vi "Calculate Intersection Circles.vi"(6 "r2":dbl, 7 "r1":dbl, 8 "d":dbl, 9 "c":dbl, 10 "b":dbl, 11 "a":dbl) -> (0 "y2":dbl, 1 "x2":dbl, 2 "y1":dbl, 3 "x1":dbl)   [LabVIEW 2014, in "Position.lvclass"]
uses:
  Position.lvclass
panel:
  out "k":dbl
  out "p":dbl
  out "f":dbl
  out "e":dbl
  # "Usage:\n(a, b) signifies the (x, y) coordinates of circle 1 with radius r1.\n(c, d) signifies the (x, y) coordinates of circle 2 with radius r2.\n\nThe VI will return 4 values:\n- (x, y) coordinates where / if the circles intersect, as x1 and y1.\n- (x, y) coordinates where / if the circles intersect secondly, as x2 and y2.\n\nImportant: if the circles do not intersect 'NaN' will be returned"
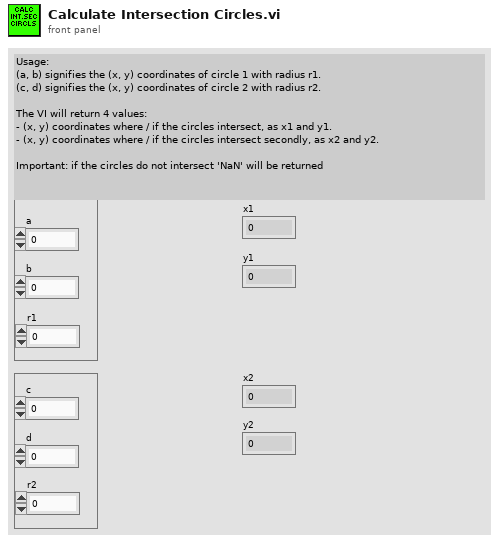
[diagram p1: front panel]
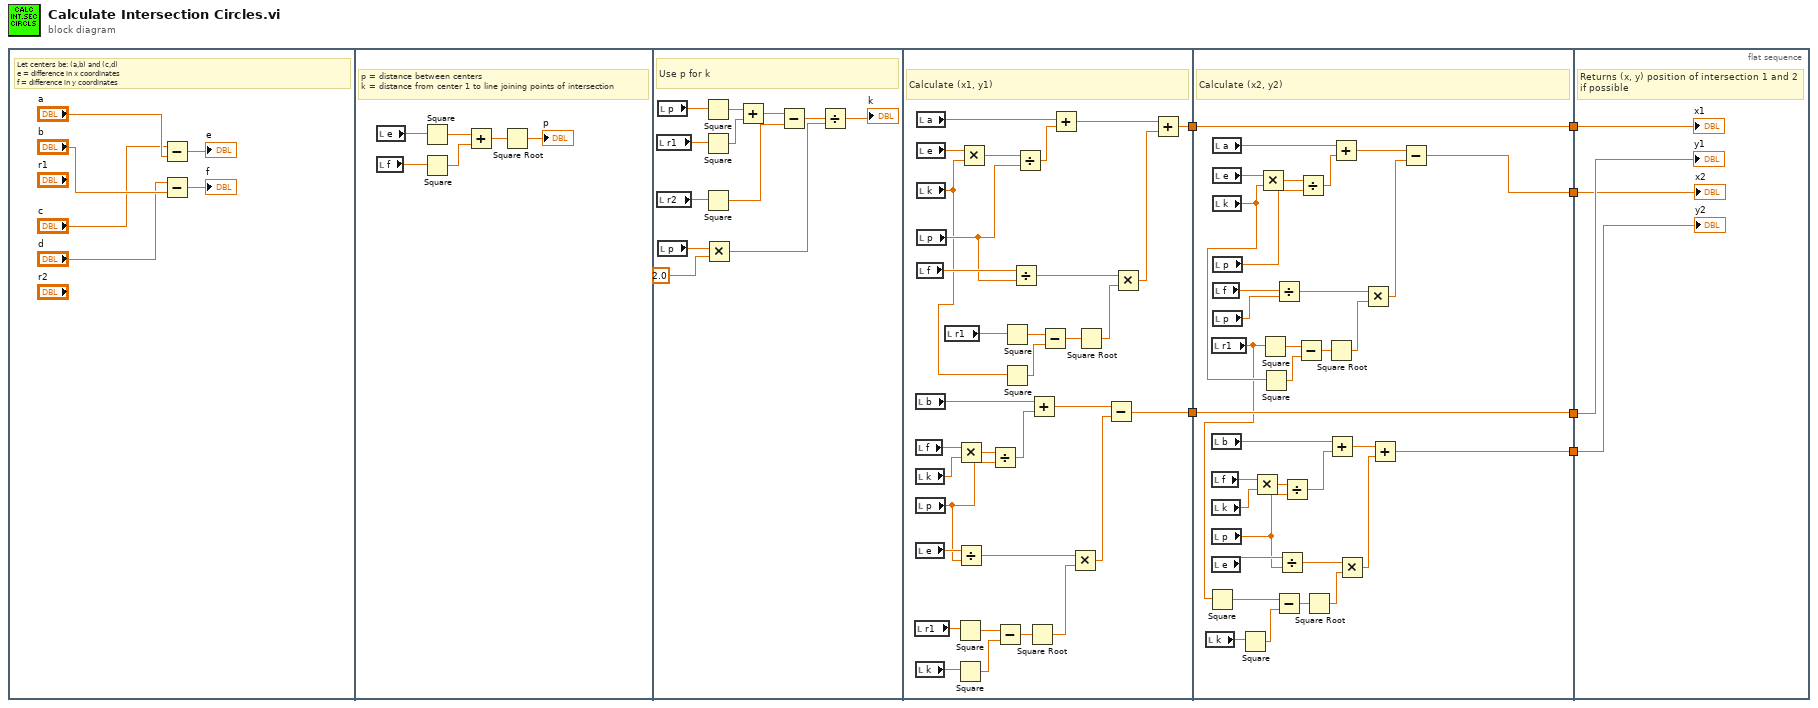
[diagram p0: block diagram]
diagram:
  n1 = flat-sequence {
    tunnel: [w32] -> w6
    tunnel: [w31] -> w4
    tunnel: w6 -> [w98]
    tunnel: [w98] -> w5
    tunnel: w4 -> [w97]
    tunnel: [w97] -> w3
    tunnel: [w83] -> w2
    tunnel: [w66] -> w1
    tunnel: w5 -> [w102]
    tunnel: w3 -> [w101]
    tunnel: w2 -> [w100]
    tunnel: w1 -> [w99]
    frame #0 {
      # "Let centers be: (a,b) and (c,d)\ne = difference in x coordinates\nf = difference in y coordinates"
      n2 = Subtract(x="c", y="a") -> (x-y=→"e":dbl)
      n3 = Subtract(x="d", y="b") -> (x-y=→"f":dbl)
    }
    frame #1 {
      # "p = distance between centers\nk = distance from center 1 to line joining points of intersection"
      n4 = local read "e"() -> (w13:dbl)
      n5 = local read "f"() -> (w14:dbl)
      n6 = Square(x=w13) -> (x^2=w15:dbl)
      n7 = Square(x=w14) -> (x^2=w16:dbl)
      n8 = Add(x=w15, y=w16) -> (x+y=w17:dbl)
      n9 = Square Root(x=w17) -> (sqrt(x)=→"p":dbl)
    }
    frame #2 {
      # "Use p for k"
      n10 = local read "r1"() -> (w28:dbl)
      n11 = local read "r2"() -> (w26:dbl)
      n12 = local read "p"() -> (w30:dbl)
      n13 = local read "p"() -> (w21:dbl)
      n14 = Square(x=w30) -> (x^2=w29:dbl)
      n15 = Square(x=w28) -> (x^2=w27:dbl)
      n16 = Square(x=w26) -> (x^2=w24:dbl)
      n17 = Multiply(x=w21, y=2.0) -> (x*y=w20:dbl)
      n18 = Add(x=w29, y=w27) -> (x+y=w25:dbl)
      n19 = Subtract(x=w25, y=w24) -> (x-y=w23:dbl)
      n20 = Divide(x=w23, y=w20) -> (x/y=→"k":dbl)
    }
    frame #3 {
      # "Calculate (x1, y1)"
      n21 = local read "r1"() -> (w42:dbl)
      n22 = local read "b"() -> (w51:dbl)
      n23 = local read "f"() -> (w50:dbl)
      n24 = local read "k"() -> (w49:dbl)
      n25 = local read "p"() -> (w44:dbl)
      n26 = local read "e"() -> (w45:dbl)
      n27 = local read "k"() -> (w41:dbl)
      n28 = local read "a"() -> (w61:dbl)
      n29 = local read "e"() -> (w63:dbl)
      n30 = local read "k"() -> (w55:dbl)
      n31 = local read "p"() -> (w58:dbl)
      n32 = local read "f"() -> (w59:dbl)
      n33 = local read "r1"() -> (w56:dbl)
      n34 = Square(x=w42) -> (x^2=w40:dbl)
      n35 = Square(x=w41) -> (x^2=w39:dbl)
      n36 = Multiply(x=w50, y=w49) -> (x*y=w48:dbl)
      n37 = Divide(x=w45, y=w44) -> (x/y=w43:dbl)
      n38 = Multiply(x=w63, y=w55) -> (x*y=w62:dbl)
      n39 = Divide(x=w48, y=w44) -> (x/y=w47:dbl)
      n40 = Subtract(x=w40, y=w39) -> (x-y=w38:dbl)
      n41 = Square(x=w56) -> (x^2=w54:dbl)
      n42 = Square(x=w55) -> (x^2=w53:dbl)
      n43 = Divide(x=w59, y=w58) -> (x/y=w35:dbl)
      n44 = Divide(x=w62, y=w58) -> (x/y=w60:dbl)
      n45 = Square Root(x=w38) -> (sqrt(x)=w37:dbl)
      n46 = Add(x=w51, y=w47) -> (x+y=w46:dbl)
      n47 = Subtract(x=w54, y=w53) -> (x-y=w52:dbl)
      n48 = Add(x=w61, y=w60) -> (x+y=w57:dbl)
      n49 = Multiply(x=w43, y=w37) -> (x*y=w36:dbl)
      n50 = Square Root(x=w52) -> (sqrt(x)=w34:dbl)
      n51 = Subtract(x=w46, y=w36) -> (x-y=w31:dbl)
      n52 = Multiply(x=w35, y=w34) -> (x*y=w33:dbl)
      n53 = Add(x=w57, y=w33) -> (x+y=w32:dbl)
    }
    frame #4 {
      # "Calculate (x2, y2)"
      n54 = local read "k"() -> (w72:dbl)
      n55 = local read "r1"() -> (w73:dbl)
      n56 = Square(x=w73) -> (x^2=w71:dbl)
      n57 = local read "b"() -> (w82:dbl)
      n58 = local read "f"() -> (w81:dbl)
      n59 = local read "k"() -> (w80:dbl)
      n60 = local read "p"() -> (w75:dbl)
      n61 = local read "e"() -> (w76:dbl)
      n62 = local read "a"() -> (w96:dbl)
      n63 = local read "e"() -> (w65:dbl)
      n64 = local read "k"() -> (w89:dbl)
      n65 = local read "p"() -> (w94:dbl)
      n66 = local read "f"() -> (w91:dbl)
      n67 = local read "p"() -> (w90:dbl)
      n68 = Square(x=w72) -> (x^2=w70:dbl)
      n69 = Multiply(x=w81, y=w80) -> (x*y=w79:dbl)
      n70 = Multiply(x=w65, y=w89) -> (x*y=w95:dbl)
      n71 = Square(x=w73) -> (x^2=w88:dbl)
      n72 = Square(x=w89) -> (x^2=w87:dbl)
      n73 = Divide(x=w91, y=w90) -> (x/y=w85:dbl)
      n74 = Subtract(x=w71, y=w70) -> (x-y=w69:dbl)
      n75 = Divide(x=w76, y=w75) -> (x/y=w74:dbl)
      n76 = Divide(x=w79, y=w75) -> (x/y=w78:dbl)
      n77 = Subtract(x=w88, y=w87) -> (x-y=w86:dbl)
      n78 = Divide(x=w95, y=w94) -> (x/y=w93:dbl)
      n79 = Square Root(x=w69) -> (sqrt(x)=w68:dbl)
      n80 = Square Root(x=w86) -> (sqrt(x)=w64:dbl)
      n81 = Add(x=w82, y=w78) -> (x+y=w77:dbl)
      n82 = Add(x=w96, y=w93) -> (x+y=w92:dbl)
      n83 = Multiply(x=w74, y=w68) -> (x*y=w67:dbl)
      n84 = Multiply(x=w85, y=w64) -> (x*y=w84:dbl)
      n85 = Add(x=w77, y=w67) -> (x+y=w66:dbl)
      n86 = Subtract(x=w92, y=w84) -> (x-y=w83:dbl)
    }
    frame #5 {
      # "Returns (x, y) position of intersection 1 and 2 if possible"
      "x1" <- w102
      "y1" <- w101
      "x2" <- w100
      "y2" <- w99
    }
  }
